vi "util.file.ini.vi"(6 "Operation(Read)":enum16{"Read", "Write"}(ring), 7 "Section":T1, 8 "error in":errorcluster, 9 "values":string[](array[string]), 10 "keys":T2[](array[typedef])) -> (0 "error out":errorcluster, 1 "values":string[](array[string]), 2 "found?":bool)   [LabVIEW 2024]
uses:
  controls/ini-key.ctl
  controls/typeIniFileSection.ctl
  controls/typePathSelector.ctl
  <vilib>/Utility/error.llb/Clear Errors.vi
  <vilib>/Utility/libraryn.llb/Create Directory Recursive.vi
  <vilib>/Utility/config.llb/Read Key (String).vi
  <vilib>/Utility/config.llb/Write Key (String).vi
  <vilib>/Utility/config.llb/NI_LVConfig.lvlib
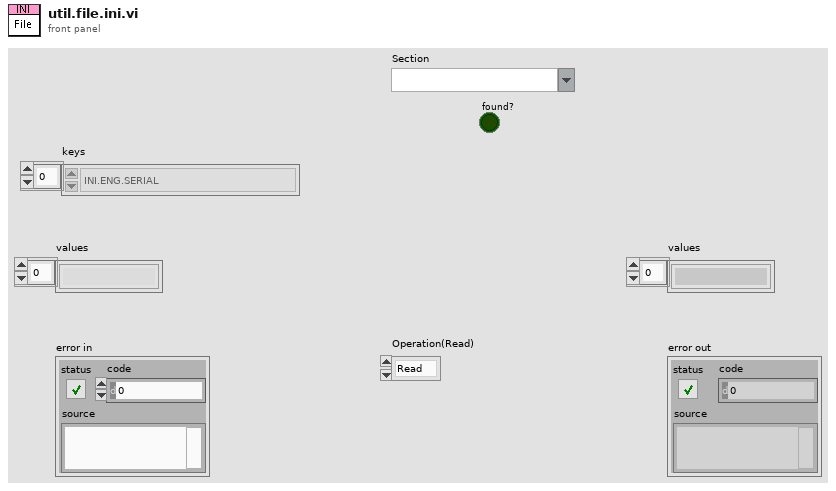
[diagram p1: front panel]
types:
  T1 = typedef "typeIniFileSection.ctl" = string
  T2 = typedef "ini-key.ctl" = enum16{"INI.PROJECT_NAME", "INI.ENV", "INI.ENG.SERIAL", "INI.ENG.INTERVAL_MS", "INI.LOCAL.LONGITUDE", "INI.LOCAL.LATITUDE", "INI.LOCAL.TIMEZONE"}
  T3 = typedef "typePathSelector.ctl" = enum16{"DIR_PROCS", "DIR_CONFIG", "DIR_TEMPLATE", "DIR_IO_FILE", "DIR_RECORD", "DIR_LOG", "DIR_RUNTIME", "DIR_PRESET", "DIR_INI"}
  T4 = typedef "NI_LVConfig.lvlib/Config Data RefNum.ctl" = refnum<k1>
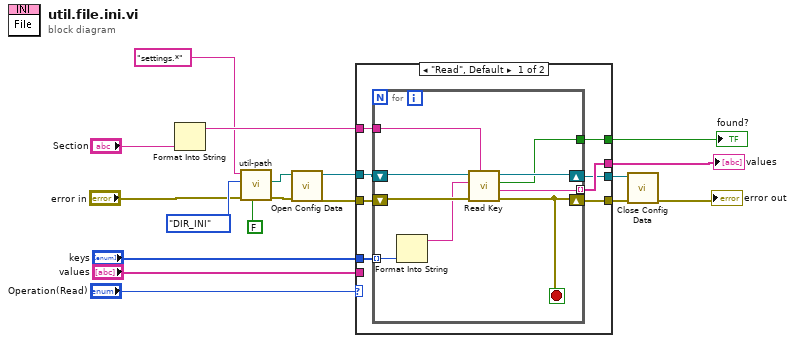
[diagram p0: block diagram]
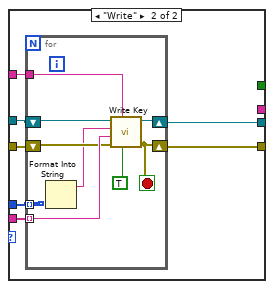
[diagram p2: hidden frame]
diagram:
  n1 = Format Into String("Section") -> (resulting string=w4:string)  [unwired: 3 in, 1 out]
  n2 = call "util-path.vi"("Create Folders?(F)"=FALSE, "error in"="error in", "Selected Folder (PROCS)"=typePathSelector."DIR_INI" ("Selected Folder (PROCEDURE_DIR)"), "append path (ie. folder\\filename.*)"="settings.*") -> ("error out"=w16:errorcluster, "SelectedPath"=w14:path)  [unwired: 3 in, 3 out]
  n3 = call <vilib>:"Open Config Data.vi"("error in (no error)"=w16, "configuration file path"=w14) -> ("error out"=w15:errorcluster, "refnum"=w13:T4)  [unwired: 7 in, 1 out]
  n4 = case shown="\"Read\", Default" "Operation(Read)" {
    tunnel: "values" -> [_ w42]
    tunnel: "keys" -> [w26 w41]
    tunnel: w15 -> [w25 w40]
    tunnel: w4 -> [w24 w39]
    tunnel: w13 -> [w23 w38]
    tunnel: [w22 _] -> w9
    tunnel: [w21 w37] -> w8
    tunnel: [w20 w36] -> w7
    tunnel: [w19 _] -> w1
    frame "Read", Default {
      n5 = for {
        tunnel: w24 -> [w33]
        shift-right: [w34] -> w20
        shift-left: w23 -> [w35]
        shift-right: [w31] -> w21
        shift-left: w25 -> [w32]
        tunnel: w26 -> [w28] mode=indexing
        tunnel: [w30] -> w22 mode=indexing
        tunnel: [w27] -> w19
        stop <- w31 stop-if-true
        n6 = Format Into String(w28) -> (resulting string=w29:string)  [unwired: 3 in, 1 out]
        n7 = call-poly <vilib>:"Read Key.vi"("section"=w33, "error in (no error)"=w32, "key"=w29, "refnum"=w35) -> ("error out"=w31:errorcluster, "value"=w30:string, "found?"=w27:bool, "refnum out"=w34:T4)  [unwired: 4 in]
      }
    }
    frame "Write" {
      n8 = for {
        tunnel: w39 -> [w45]
        shift-right: [w50] -> w36
        shift-left: w38 -> [w51]
        shift-right: [w48] -> w37
        shift-left: w40 -> [w47]
        tunnel: w41 -> [w43] mode=indexing
        tunnel: w42 -> [w49] mode=indexing
        stop <- w48 stop-if-true
        n9 = Format Into String(w43) -> (resulting string=w44:string)  [unwired: 3 in, 1 out]
        n10 = call-poly <vilib>:"Write Key.vi"("write raw string? (F)"=TRUE, "section"=w45, "error in (no error)"=w47, "value"=w49, "key"=w44, "refnum"=w51) -> ("error out"=w48:errorcluster, "refnum out"=w50:T4)  [unwired: 3 in, 1 out]
      }
    }
  }
  "values" <- w9
  "found?" <- w1
  n11 = call <vilib>:"Close Config Data.vi"("error in (no error)"=w8, "refnum"=w7) -> ("error out"=→"error out":errorcluster)  [unwired: 8 in, 1 out]
